vi "_U64Out.vi"(2 "Data":u64, 3 "Refnum in":refnum<k21>) -> ()   [LabVIEW 2018]
uses:
  <vilib>/rvi/DataTransferAndStorage/Container/Common/niFpgaContainerExecOnDevCompGetState.vi
  <vilib>/rvi/Emulation/niFpgaEmulationIsFPGAContextNoSignature.vi
  <vilib>/rvi/Emulation/niFpgaSctlEmulationGetInTimedLoop.vi
  <vilib>/rvi/errors/niFpgaSetErrorForExecOnDevCompSimple.vi
  <vilib>/rvi/eio/common/nirviEmuReportErrorAndStop.vi
  <vilib>/rvi/DataTransferAndStorage/Container/Common/niFpgaContainerGetUniqueNameForEmu.vi
  <vilib>/rvi/FIFO/Fifo_Resource/nirvififoEmulationSetSize.vi
  <vilib>/rvi/FIFO/Fifo_Resource/nirviFifoEmulationQueueMgr.vi
  <instcachedir>/0/nirviFifoEmulationQueueMgr_E5CAEC123FF24DC58D834DCA3CDAA9B5.lvgen/nirviFifoEmulationQueueMgr_E5CAEC123FF24DC58D834DCA3CDAA9B5_001.vi
  <vilib>/rvi/FIFO/Fifo_Resource/nirvififoEmulationDetermineInputValidOut.vi
  <vilib>/rvi/FIFO/Fifo_Resource/nirvififoEmulationCreateLock.vi
  <vilib>/rvi/Emulation/niFpgaProcessEmulError.vi
  <vilib>/rvi/FIFO/Fifo_Resource/nirvififoEmulationObtainLock.vi
  <vilib>/rvi/FIFO/Fifo_Resource/nirvififoEmulationReleaseLock.vi
  <vilib>/rvi/occurrence/nirviWaitOnOccurrenceBase.vi
  <vilib>/rvi/errors/nirviReportUnexpectedCaseInternalError.vi
  <vilib>/rvi/errors/nirviReportUnexpectedCaseInternalError (U32).vi
  <vilib>/Utility/error.llb/Clear Errors.vi
  <vilib>/rvi/interface/RandomDataEmulation/niFpgaRandomDataHandleErrors.vi
  <vilib>/rvi/DataTransferAndStorage/Container/XNode/niFpgaContainer.xnode
  <vilib>/rvi/FIFO/Fifo_Resource/niFpgaFifoEmulationRefIn.vi
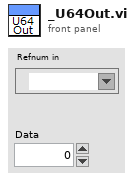
[diagram p1: front panel]
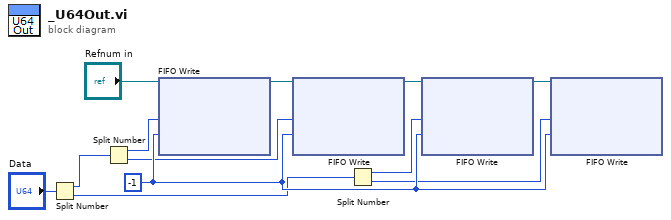
[diagram p0: block diagram]
diagram:
  w12 = -1 ("Timeout")
  n1 = Split Number(x="Data") -> (hi(x)=w2:u32, lo(x)=w3:u32)
  n2 = Split Number(x=w2) -> (hi(x)=w5:u16, lo(x)=w9:u16)
  n3 = xnode ("FIFO Write")("Element"=w5, "Timeout"=w12, "FIFO In"="Refnum in") -> ("FIFO Out"=w6:refnum<k21>)  [unwired: 1 out]
  n4 = xnode ("FIFO Write")("Element"=w9, "Timeout"=w12, "FIFO In"=w6) -> ("FIFO Out"=w7:refnum<k21>)  [unwired: 1 out]
  n5 = Split Number(x=w3) -> (hi(x)=w10:u16, lo(x)=w11:u16)
  n6 = xnode ("FIFO Write")("Element"=w10, "Timeout"=w12, "FIFO In"=w7) -> ("FIFO Out"=w8:refnum<k21>)  [unwired: 1 out]
  n7 = xnode ("FIFO Write")("Element"=w11, "Timeout"=w12, "FIFO In"=w8) -> ()  [unwired: 2 out]
